vi "13- Remove leading zeros in string.vi"() -> ()   [LabVIEW 2019]
panel:
  out "Output string":string
  in  "Input string":string
  # "REMOVE LEADING ZEROS FROM INPUT STRING"
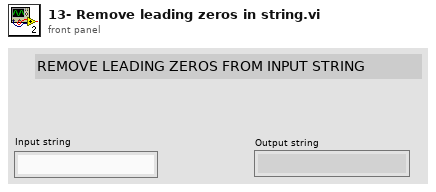
[diagram p1: front panel]
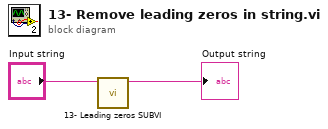
[diagram p0: block diagram]
diagram:
  n1 = call "13- Leading zeros SUBVI.vi"("Input string"="Input string") -> ("String"=→"Output string":string)  [unwired: 10 in]
